vi "Write TimeN.vi"(8 "error in (no error)":errorcluster, 10 "TimeN":refnum<notifier>, 11 "SquareBattle Arena in":refnum<class "SquareBattle Arena.lvclass">) -> (0 "error out":errorcluster, 3 "SquareBattle Arena out":refnum<class "SquareBattle Arena.lvclass">)   [LabVIEW 2014, in "SquareBattle Arena.lvlib" / "SquareBattle Arena.lvclass"]
uses:
  SquareBattle Arena.lvclass
  SquareBattle Arena.lvclass/SquareBattle Arena.ctl
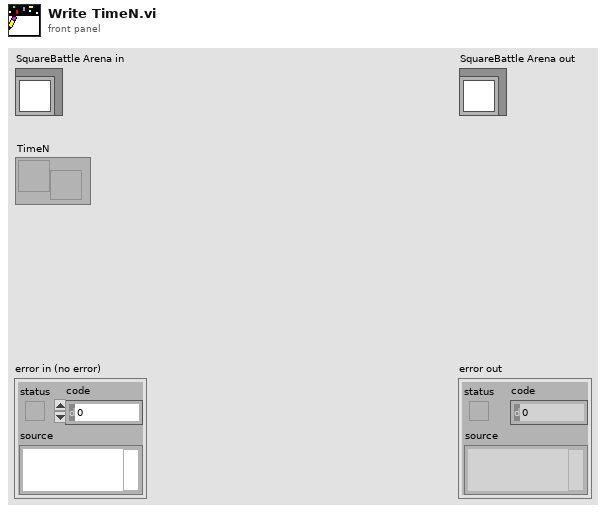
[diagram p1: front panel]
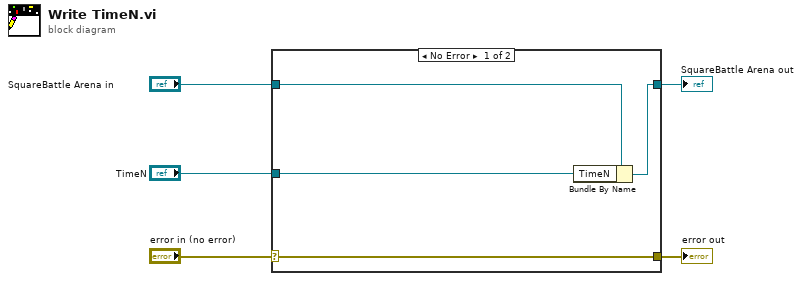
[diagram p0: block diagram]
diagram:
  n1 = case shown="No Error" "error in (no error)" {
    selector: "error in (no error)" -> [w9 w10]
    tunnel: [w9 w10] -> w4
    tunnel: [w7 w11] -> w2
    tunnel: "SquareBattle Arena in" -> [w8 w11]
    tunnel: "TimeN" -> [w6 _]
    frame No Error {
      n2 = Bundle By Name(cluster=w8, "TimeN"=w6) -> (w7:refnum<class "SquareBattle Arena.lvclass">)
    }
    frame Error {
    }
  }
  "error out" <- w4
  "SquareBattle Arena out" <- w2
